vi "Ref Emergency.vi"(8 "error in (no error)":errorcluster, 11 "Sim Display Console Actor in":refnum<class "Sim Display Console Actor.lvclass">) -> (0 "error out":errorcluster, 2 "Emergency":refnum<vi>, 3 "Sim Display Console Actor out":refnum<class "Sim Display Console Actor.lvclass">)   [LabVIEW 2019, in "Simulated Display Console Actor.lvlib" / "Sim Display Console Actor.lvclass"]
uses:
  Sim Display Console Actor.lvclass
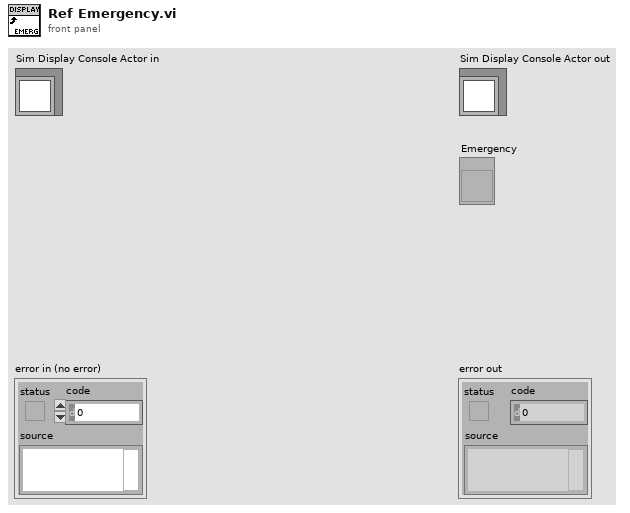
[diagram p1: front panel]
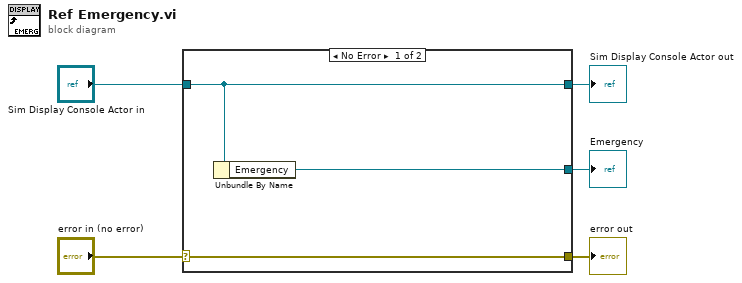
[diagram p0: block diagram]
diagram:
  n1 = case shown="No Error" "error in (no error)" {
    selector: "error in (no error)" -> [w8 w9]
    tunnel: [w8 w9] -> w4
    tunnel: [w7 w10] -> w2
    tunnel: "Sim Display Console Actor in" -> [w7 w10]
    tunnel: [w6 _] -> w1
    frame No Error {
      n2 = Unbundle By Name(w7) -> ("Emergency"=w6:refnum<vi>)
    }
    frame Error {
    }
  }
  "error out" <- w4
  "Sim Display Console Actor out" <- w2
  "Emergency" <- w1
